vi "onExportResults.vi"(8 "error in (no error)":errorcluster, 11 "Pips.TestResults in":refnum<class "Pips.TestResults.lvclass">) -> (0 "error out":errorcluster, 3 "Pips.TestResults out":refnum<class "Pips.TestResults.lvclass">)   [LabVIEW 2021, in "Banana.Caraya.lvlib" / "Pips.TestResults.lvclass"]
uses:
  Pips.TestResults.lvclass
  Pips.TestResults.lvclass/Pips.TestResults.ctl
  Bananas/Datastore.Dictionaries/Datastore.Dictionaries.lvclass
  <vilib>/Utility/Data Type/NI_Data Type.lvlib
  <vilib>/LabVIEW Open Source Project/Data Manipulation/Variant/OpenVariant.lvlib
panel:
  in  "Other":i32(listbox)
  in  "Coverage":i32(listbox)
  in  "Summary":i32(listbox)
  out "Titles":string[](array[string])
  out "Pictures":picture[](array[picture])
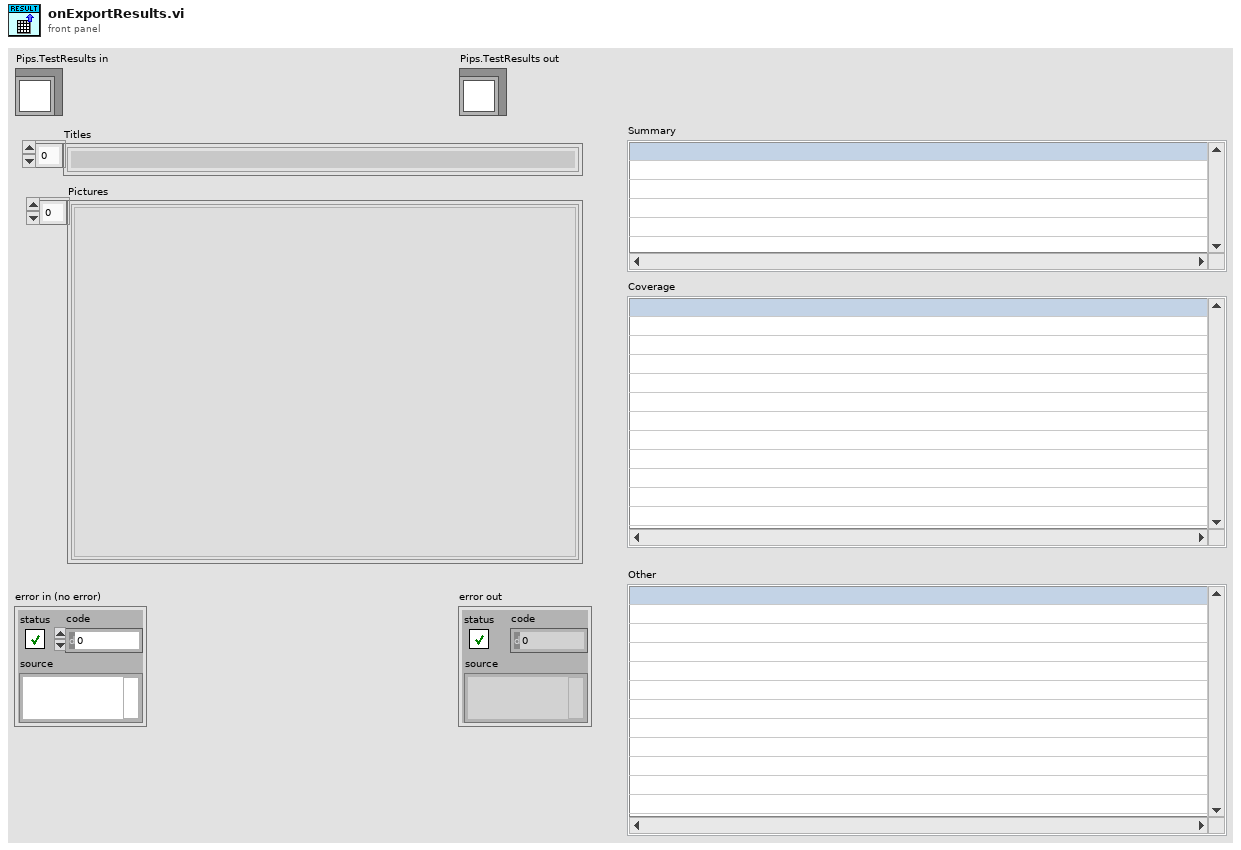
[diagram p1: front panel]
types:
  T1 = cluster{"Images":map{string, picture}, "Summary":map{string, string}, "Coverage":map{string, string}, "Other":map{string, string}}
  T2 = typedef "NI_Data Type.lvlib/Data Type.ctl" = enum8{"Invalid Type", "Void", "I8", "I16", "I32", "I64", "U8", "U16", "U32", "U64", "Single Float", "Double Float", "Extended Float", "Single Complex", "Double Complex", "Extended Complex", "Enum U8", "Enum U16", "Enum U32", "Enum U64", "Single Float With Unit", "Double Float With Unit", "Extended Float With Unit", "Single Complex with Unit", "Double Complex with Unit", "Extended Complex with Unit", "Boolean", "String", "Path", "Picture", "Tag", "Array", "Cluster", "Variant", "LV Variant", "Waveform", "Timestamp", "Digital Waveform", "Digital Data", "ExpressData", "Refnum", "External Data", "VI", "Poly VI", "LabVIEW Class Instance", "Fixed Point", "Set Collection", "Map Collection"}
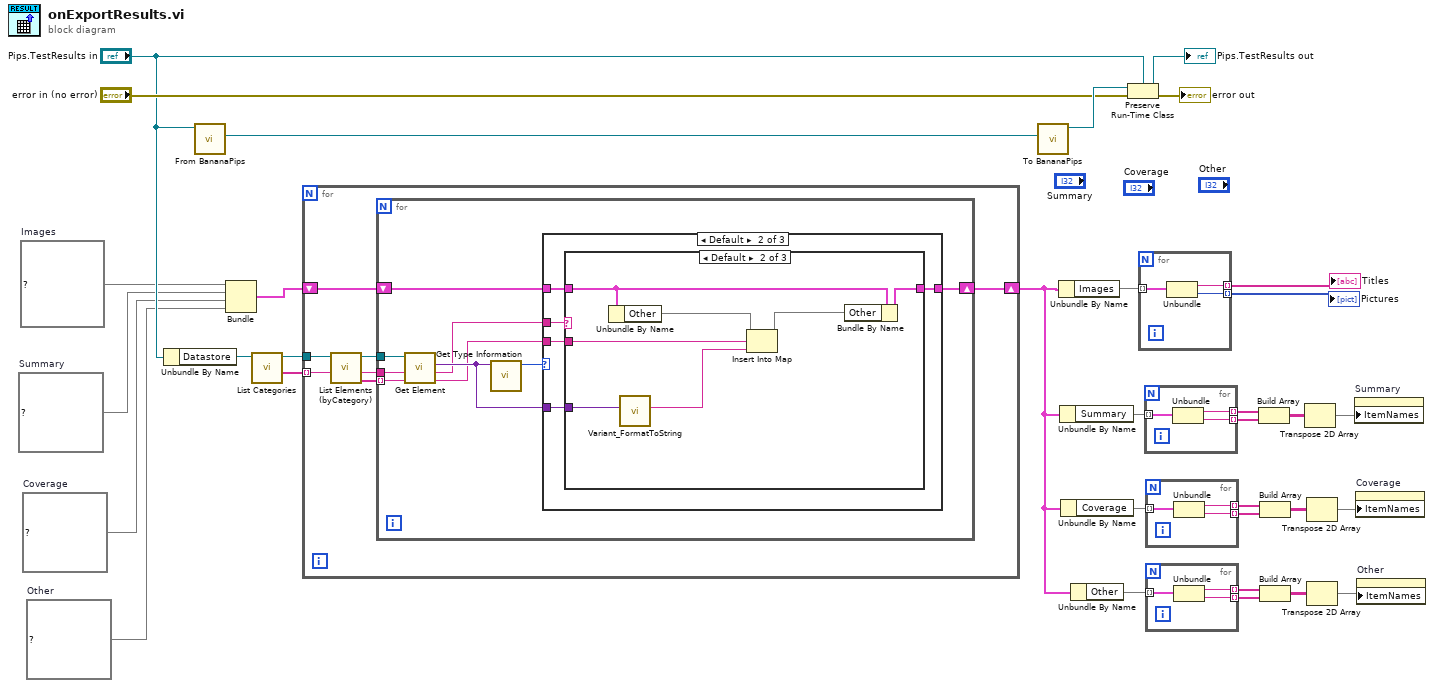
[diagram p0: block diagram]
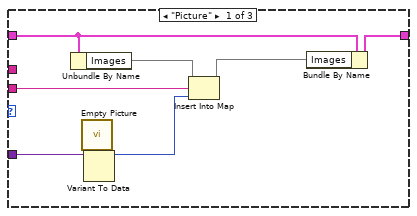
[diagram p2: hidden frame]
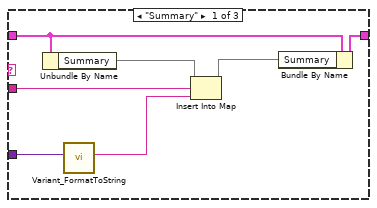
[diagram p3: hidden frame]
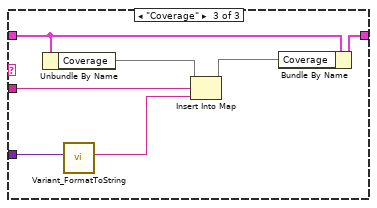
[diagram p4: hidden frame]
diagram:
  w2 = map{string, string} {}  # Other
  w14 = map{string, string} {}  # Coverage
  w19 = map{string, string} {}  # Summary
  w24 = map{string, picture} {}  # Images
  n1 = Unbundle By Name("Pips.TestResults in") -> ("Datastore"=w25:refnum<class "Datastore.Dictionaries.lvclass">)
  n2 = call "From BananaPips.vi"("Pips.TestResults"="Pips.TestResults in") -> ("Test Result"=w29:refnum<class "Test Result.lvclass">)  [unwired: 10 in]
  n3 = Bundle("Images"=w24, "Summary"=w19, "Coverage"=w14, "Other"=w2) -> (w23:T1)  [unwired: 1 in]
  n4 = call "List Categories.vi"("Datastore.Dictionaries in"=w25) -> ("categories"=w27:string[], "Datastore.Dictionaries"=w26:refnum<class "Datastore.Dictionaries.lvclass">)  [unwired: 9 in]
  n5 = for {
    tunnel: w26 -> [w39]
    tunnel: w27 -> [w36] mode=indexing
    shift-right: [w34] -> w3
    shift-left: w23 -> [w35]
    n6 = call "List Elements (byCategory).vi"("category"=w36, "Datastore.Dictionaries in"=w39) -> ("elements"=w38:string[], "category dup"=w37:string, "Datastore.Dictionaries"=w40:refnum<class "Datastore.Dictionaries.lvclass">)  [unwired: 6 in, 1 out]
    n7 = for {
      tunnel: w40 -> [w49]
      tunnel: w38 -> [w48] mode=indexing
      tunnel: w37 -> [w47]
      shift-right: [w44] -> w34
      shift-left: w35 -> [w45]
      n8 = call "Get Element.vi"("element"=w48, "category"=w47, "Datastore.Dictionaries in"=w49) -> ("element dup"=w42:string, "category dup"=w41:string, "Value"=w43:variant)  [unwired: 4 in, 2 out]
      n9 = call <vilib>:"Get Type Information.vi"("variant"=w43) -> ("type"=w46:T2)  [unwired: 6 in, 4 out]
      n10 = case shown="Default" w46 {
        tunnel: w45 -> [w57 w62 w84]
        tunnel: [w56 w61 w84] -> w44
        tunnel: w43 -> [w53 w60 _]
        tunnel: w42 -> [w50 w59 _]
        tunnel: w41 -> [_ w58 _]
        frame "Picture" {
          n11 = Unbundle By Name(w57) -> ("Images"=w54:map{string, picture})
          n12 = call "Empty Picture"() -> ("empty picture"=w52:picture)
          n13 = Variant To Data(type=w52, Variant=w53) -> (data=w51:picture)  [unwired: 1 in, 1 out]
          n14 = Insert Into Map(map in=w54, key=w50, value=w51) -> (map out=w55:map{string, picture})  [unwired: 2 out]
          n15 = Bundle By Name(cluster=w57, "Images"=w55) -> (w56:T1)
        }
        frame Default {
          n16 = case shown="Default" w58 {
            tunnel: w62 -> [w69 w76 w83]
            tunnel: [w68 w75 w82] -> w61
            tunnel: w60 -> [w64 w71 w78]
            tunnel: w59 -> [w65 w72 w79]
            frame "Summary" {
              n17 = Unbundle By Name(w69) -> ("Summary"=w66:map{string, string})
              n18 = call <vilib>:"Variant_FormatToString.vi"("Variant"=w64) -> ("Value"=w63:string)  [unwired: 10 in]
              n19 = Insert Into Map(map in=w66, key=w65, value=w63) -> (map out=w67:map{string, string})  [unwired: 2 out]
              n20 = Bundle By Name(cluster=w69, "Summary"=w67) -> (w68:T1)
            }
            frame Default {
              n21 = Unbundle By Name(w76) -> ("Other"=w73:map{string, string})
              n22 = call <vilib>:"Variant_FormatToString.vi"("Variant"=w71) -> ("Value"=w70:string)  [unwired: 10 in]
              n23 = Insert Into Map(map in=w73, key=w72, value=w70) -> (map out=w74:map{string, string})  [unwired: 2 out]
              n24 = Bundle By Name(cluster=w76, "Other"=w74) -> (w75:T1)
            }
            frame "Coverage" {
              n25 = Unbundle By Name(w83) -> ("Coverage"=w80:map{string, string})
              n26 = call <vilib>:"Variant_FormatToString.vi"("Variant"=w78) -> ("Value"=w77:string)  [unwired: 10 in]
              n27 = Insert Into Map(map in=w80, key=w79, value=w77) -> (map out=w81:map{string, string})  [unwired: 2 out]
              n28 = Bundle By Name(cluster=w83, "Coverage"=w81) -> (w82:T1)
            }
          }
        }
        frame "Void" {
        }
      }
    }
  }
  n29 = call "To BananaPips.vi"("Test Result"=w29) -> ("Pips.TestResults"=w33:refnum<class "Pips.TestResults.lvclass">)  [unwired: 10 in]
  n30 = Unbundle By Name(w3) -> ("Images"=w22:map{string, picture})
  n31 = Unbundle By Name(w3) -> ("Summary"=w18:map{string, string})
  n32 = Unbundle By Name(w3) -> ("Coverage"=w10:map{string, string})
  n33 = Unbundle By Name(w3) -> ("Other"=w7:map{string, string})
  n34 = Preserve Run-Time Class(object in=w33, error in="error in (no error)", 2:"Pips.TestResults in") -> (object out=→"Pips.TestResults out":refnum<class "Pips.TestResults.lvclass">, error out=→"error out":errorcluster)
  n35 = for {
    tunnel: w22 -> [w87] mode=indexing
    tunnel: [w86] -> w21 mode=indexing
    tunnel: [w85] -> w20 mode=indexing
    n36 = Unbundle(w87) -> ("title"=w86:string, "picture"=w85:picture)
  }
  "Pictures" <- w20
  "Titles" <- w21
  n37 = for {
    tunnel: w18 -> [w90] mode=indexing
    tunnel: [w89] -> w17 mode=indexing
    tunnel: [w88] -> w16 mode=indexing
    n38 = Unbundle(w90) -> ("name"=w89:string, "value"=w88:string)
  }
  n39 = for {
    tunnel: w10 -> [w93] mode=indexing
    tunnel: [w92] -> w11 mode=indexing
    tunnel: [w91] -> w12 mode=indexing
    n40 = Unbundle(w93) -> ("name"=w92:string, "value"=w91:string)
  }
  n41 = for {
    tunnel: w7 -> [w96] mode=indexing
    tunnel: [w95] -> w6 mode=indexing
    tunnel: [w94] -> w5 mode=indexing
    n42 = Unbundle(w96) -> ("name"=w95:string, "value"=w94:string)
  }
  n43 = Build Array(w17, w16) -> (w15:string[][])
  n44 = Build Array(w11, w12) -> (w13:string[][])
  n45 = Build Array(w6, w5) -> (w4:string[][])
  n46 = Transpose 2D Array(2D array=w15) -> (transposed array=w9:string[][])
  n47 = Transpose 2D Array(2D array=w13) -> (transposed array=w8:string[][])
  n48 = Transpose 2D Array(2D array=w4) -> (transposed array=w1:string[][])
  n49 = property on="Summary" class="MCListbox (strict)"("ItemNames"=w9) -> ()  [unwired: 2 in, 2 out]
  n50 = property on="Coverage" class="MCListbox (strict)"("ItemNames"=w8) -> ()  [unwired: 2 in, 2 out]
  n51 = property on="Other" class="MCListbox (strict)"("ItemNames"=w1) -> ()  [unwired: 2 in, 2 out]
